vi "Overlord - MAIN - STARTUP.vi"(0 "Pathfinding Settings":T1={"Movement Settings"={"Arrival Tolerance (m)"=0.05, "Closeness Threshold (m)"=0.5, "Pit Obstacle Radius (m)"=0.4, "Pit Locations"=[]}, "Dead Zone"=0.9, "Max Moves"=4.0, "Move Segment Length (m)"=0.2, "Path Cost Weights"={"Length Weight"=1.0, "Angle Weight"=0.0, "Angle Error Weight"=75.0, "Angle Error Threshold"=1.04, "Per Move Penalty"=0.25, "Closeness Weight"=3.0, "Too Short Penalty"=100.0, "Too Short Threshold"=1.75}, "Desperation - Reduction Per Attempt (Ratio)"=0.9, "Desperation - Max Attempts"=2, "Log All Move Points"=FALSE, "Intermediate Position Grids"=[{"x1"=0.0, "x2"=4.75, "resolution"=0.45}]}) -> ()   [LabVIEW 2015, in "Overlord2017.lvlib"]
doc: "Note: pathfinding settings not required. This VI can run headless. Set default values before deploying to myRIO."
uses:
  Overlord2017.lvlib
  PathfindingSettings.ctl
  MovementSettings.ctl
  PathCostWeights.ctl
  IntermediatePositionGrids.ctl
  SubVIs - Overlord2017.lvlib
  TestbenchUtils - Navigation2017.lvlib
  Navigation2017.lvlib
  <vilib>/myRIO/Common/Instrument Driver Framework/Utilities/typedefs/Analog Scaling Constants.ctl
  <vilib>/myRIO/Common/Instrument Driver Framework/Utilities/typedefs/Analog Scaling Constants List.ctl
  <vilib>/myRIO/Common/Instrument Driver Framework/myRIO v1.0/AI/typedefs/AI Channels Enum.ctl
  <vilib>/myRIO/Common/Instrument Driver Framework/myRIO v1.0/AI/typedefs/AI Channels List.ctl
  <vilib>/myRIO/Common/Instrument Driver Framework/Utilities/typedefs/Generic FPGA Reference.ctl
  <vilib>/myRIO/Common/Instrument Driver Framework/Utilities/typedefs/myRIO v1.0 Reference.ctl
  <vilib>/myRIO/Common/Instrument Driver Framework/Utilities/typedefs/Hardware Version Enum.ctl
  <vilib>/myRIO/Common/Instrument Driver Framework/Utilities/typedefs/myRIO Generic Hardware Reference.ctl
  <vilib>/myRIO/Instrument Drivers/Onboard IO/AI/typedefs/AI Reference.ctl
  <vilib>/myRIO/Instrument Drivers/Onboard IO/AI/AI.lvlib
  <vilib>/myRIO/Instrument Drivers/Onboard IO/AI/vis/Read.vi
  <vilib>/myRIO/Instrument Drivers/Onboard IO/AI/vis/myRIO AI Open.xnode
  <vilib>/myRIO/Common/Instrument Driver Framework/Utilities/vis/Is FPGA Ref Available.vi
  <vilib>/myRIO/Express VI/Onboard IO/AI/AI Express VI.xnode
  <vilib>/myRIO/Common/Instrument Driver Framework/myRIO v1.0/AI/vis/myRIO v1.1 Open AI.vi
  <vilib>/userdefined/High Color/nirio_resource_hc.ctl
  Types - Navigation2017.lvlib
panel:
  out "Battery Voltage Chart":dbl(graph)=11.904298094
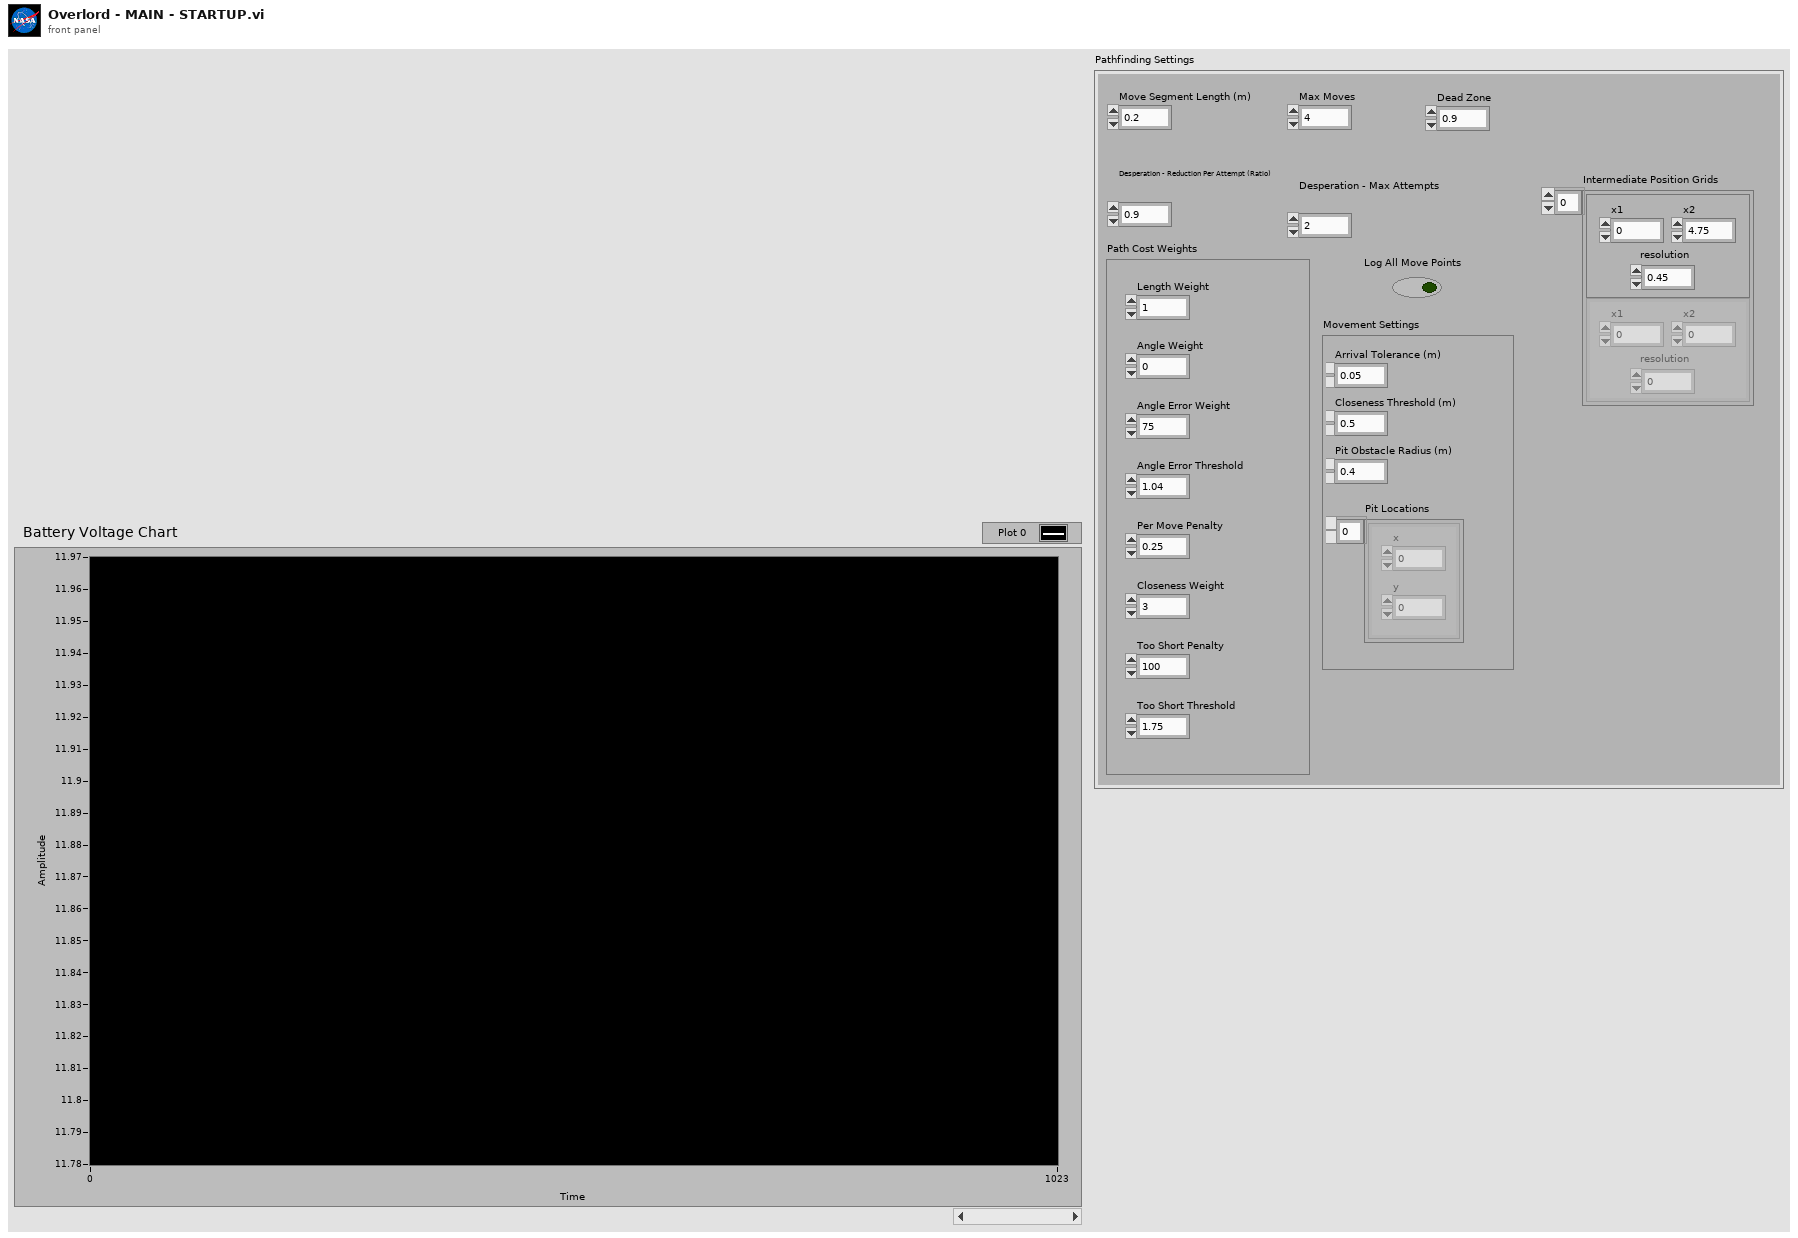
[diagram p1: front panel]
types:
  T1 = typedef "Navigation2017.lvlib/Types - Navigation2017.lvlib/PathfindingSettings.ctl" = cluster{"Movement Settings":T2, "Dead Zone":dbl, "Max Moves":dbl, "Move Segment Length (m)":dbl, "Path Cost Weights":T3, "Desperation - Reduction Per Attempt (Ratio)":dbl, "Desperation - Max Attempts":i16, "Log All Move Points":bool, "Intermediate Position Grids":T4}
  T2 = typedef "Navigation2017.lvlib/Types - Navigation2017.lvlib/MovementSettings.ctl" = cluster{"Arrival Tolerance (m)":dbl, "Closeness Threshold (m)":dbl, "Pit Obstacle Radius (m)":dbl, "Pit Locations":cluster{"x":dbl, "y":dbl}[]}
  T3 = typedef "Navigation2017.lvlib/Types - Navigation2017.lvlib/PathCostWeights.ctl" = cluster{"Length Weight":dbl, "Angle Weight":dbl, "Angle Error Weight":dbl, "Angle Error Threshold":dbl, "Per Move Penalty":dbl, "Closeness Weight":dbl, "Too Short Penalty":dbl, "Too Short Threshold":dbl}
  T4 = typedef "Navigation2017.lvlib/Types - Navigation2017.lvlib/IntermediatePositionGrids.ctl" = cluster{"x1":dbl, "x2":dbl, "resolution":dbl}[]
  T5 = typedef "AI.lvlib/AI Reference.ctl" = cluster{"myRIO Reference":T6, "AI Channels List":T10, "AI Scaling Constants List":T12}
  T6 = typedef "myRIO Generic Hardware Reference.ctl" = cluster{"myRIO Model":T7, "myRIO Hardware Reference":T8}
  T7 = typedef "Hardware Version Enum.ctl" = enum16{"Unknown", "myRIO-1900", "myRIO-1950", "roboRIO"}
  T8 = typedef "myRIO v1.0 Reference.ctl" = cluster{"Generic FPGA Reference":T9, "Allow multiple opens":bool}
  T9 = typedef "Generic FPGA Reference.ctl" = refnum<k20>
  T10 = typedef "AI Channels List.ctl" = T11[]
  T11 = typedef "AI Channels Enum.ctl" = enum16{"Not Connected", "AudioIn/Left", "AudioIn/Right", "C/AI0", "C/AI1", "A/AI0", "A/AI1", "A/AI2", "A/AI3", "B/AI0", "B/AI1", "B/AI2", "B/AI3", "AI/AI0", "AI/AI1", "AI/AI2", "AI/AI3"}
  T12 = typedef "Analog Scaling Constants List.ctl" = T13[]
  T13 = typedef "Analog Scaling Constants.ctl" = cluster{"LSB Weight (Volts)":dbl, "Offset (Volts)":dbl, "Signed?":bool}
  T14 = typedef "nirio_resource_hc.ctl" = tag
  T15 = enum16{"Spin and Move To Mining Area", "Move To Collector Trough", "Move To Mining Area"}
  T16 = typedef "Navigation2017.lvlib/TestbenchUtils - Navigation2017.lvlib/LocalizationStatus.ctl" = cluster{"x":dbl, "y":dbl, "angle":dbl, "valid":bool, "lastUpdatedTime":dbl}
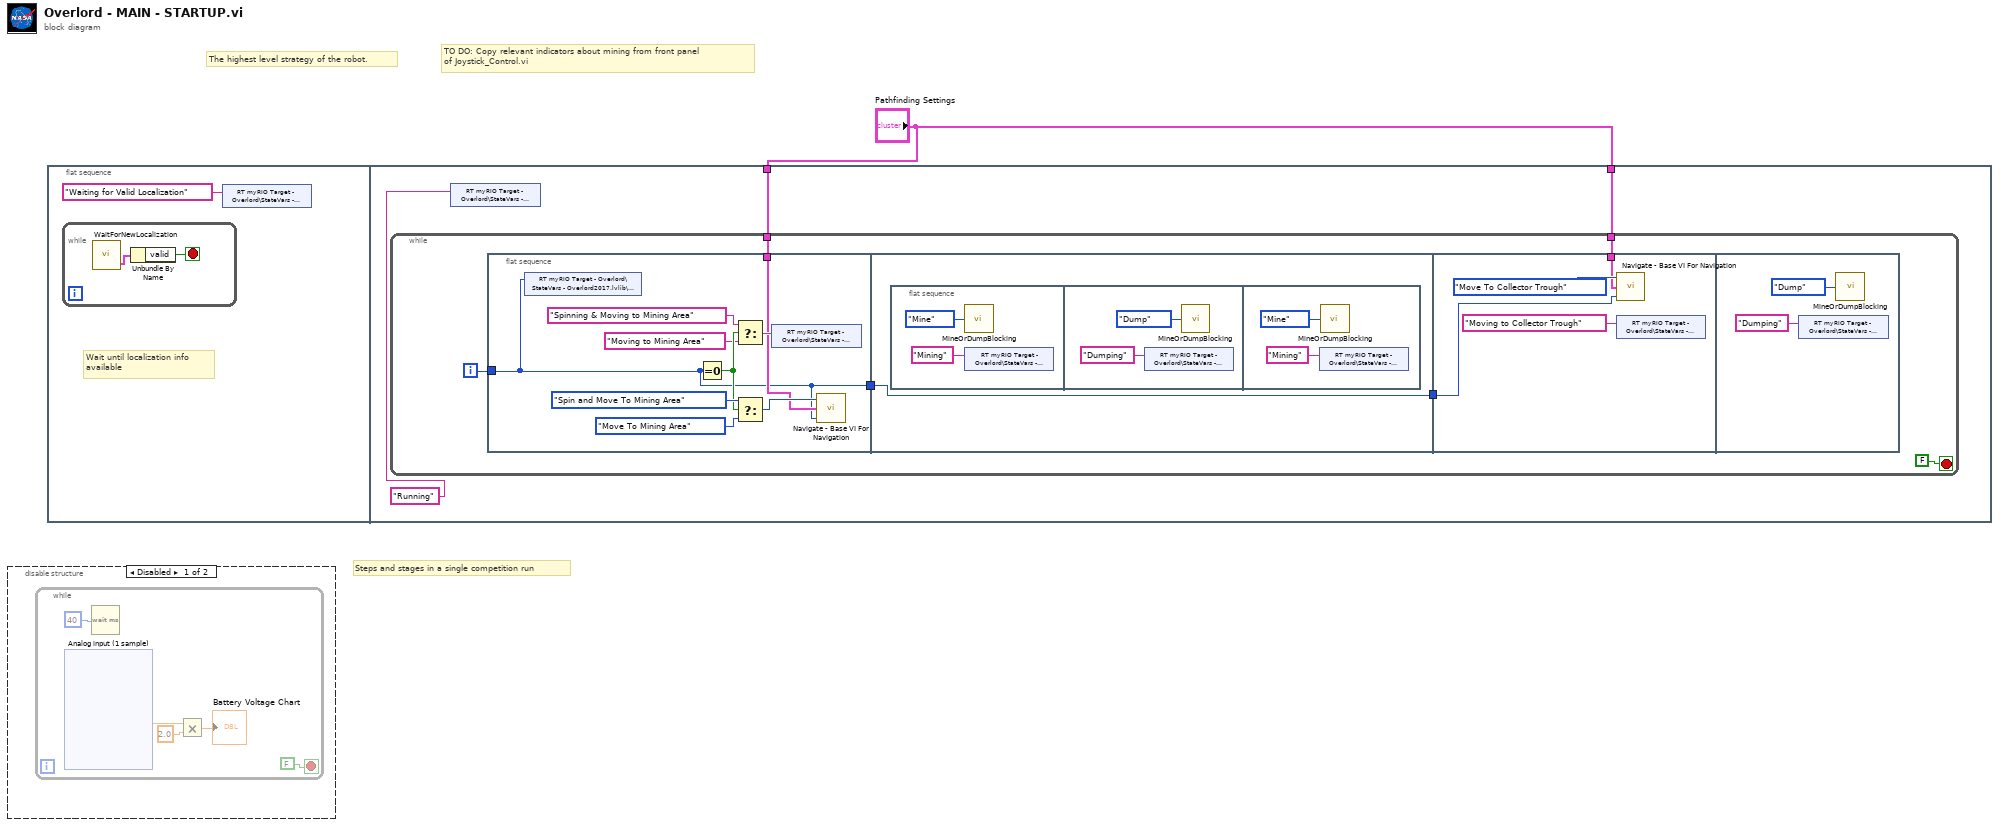
[diagram p0: block diagram]
diagram:
  # "The highest level strategy of the robot."
  # "Steps and stages in a single competition run"
  # "TO DO: Copy relevant indicators about mining from front panel\nof Joystick_Control.vi"
  n1 = disable-structure shown="Disabled" {
    frame Disabled {
      n2 = while {
        stop <- FALSE stop-if-true
        n3 = xnode "Analog input (1 sample)"() -> ("C/AI0 (AI0)"=w3:dbl)  [unwired: 1 in, 1 out]
        n4 = Wait (ms)(milliseconds to wait=u32 40) -> ()  [unwired: 1 out]
        n5 = Multiply(x=w3, y=2.0) -> (x*y=→"Battery Voltage Chart":dbl)
      }
    }
    frame Enabled {
    }
  }
  n6 = flat-sequence {
    tunnel: "Pathfinding Settings" -> [w48]
    tunnel: "Pathfinding Settings" -> [w47]
    frame #0 {
      # "Wait until localization info\navailable"
      n7 = while {
        stop <- w46 stop-if-true
        n8 = call "WaitForNewLocalization.vi"() -> ("Localization Status"=w45:T16)  [unwired: 1 out]
        n9 = Unbundle By Name(w45) -> ("valid"=w46:bool)
      }
      n10 = shared-variable "RT myRIO Target - Overlord\\StateVars - Overlord2017.lvlib\\CurrStage"("Waiting for Valid Localization" ("CurrStage")) -> ()  [unwired: 1 in, 1 out]
    }
    frame #1 {
      n11 = while {
        tunnel: w48 -> [w53]
        tunnel: w47 -> [w52]
        i -> [w55]
        stop <- FALSE stop-if-true
        n12 = flat-sequence {
          tunnel: w55 -> [w56]
          tunnel: w53 -> [w57]
          tunnel: [w56] -> w51
          tunnel: w51 -> [w65]
          tunnel: [w65] -> w50
          tunnel: w52 -> [w73]
          tunnel: w50 -> [w72]
          frame #0 {
            n13 = shared-variable "RT myRIO Target - Overlord\\StateVars - Overlord2017.lvlib\\CurrMiningRun"(w56) -> ()  [unwired: 1 in, 1 out]
            n14 = Equal To 0?(x=w56) -> (x = 0?=w59:bool)
            n15 = Select(t="Spinning & Moving to Mining Area" ("CurrStage"), s=w59, f="Moving to Mining Area") -> (s? t:f=w61:string)
            n16 = Select(t=T15."Spin and Move To Mining Area" ("Move Type"), s=w59, f=T15."Move To Mining Area") -> (s? t:f=w62:T15)
            n17 = shared-variable "RT myRIO Target - Overlord\\StateVars - Overlord2017.lvlib\\CurrStage"(w61) -> ()  [unwired: 1 in, 1 out]
            n18 = call "Navigate - Base VI For Navigation.vi"("Curr Mining Run"=w56, "Pathfinding Settings"=w57, "Move Type"=w62) -> ()  [unwired: 1 in]
          }
          frame #1 {
            n19 = flat-sequence {
              frame #0 {
                n20 = call "MineOrDumpBlocking.vi"("Action"=enum16{"Dump", "Mine"}."Mine") -> ()
                n21 = shared-variable "RT myRIO Target - Overlord\\StateVars - Overlord2017.lvlib\\CurrStage"("Mining" ("CurrStage")) -> ()  [unwired: 1 in, 1 out]
              }
              frame #1 {
                n22 = shared-variable "RT myRIO Target - Overlord\\StateVars - Overlord2017.lvlib\\CurrStage"("Dumping" ("CurrStage")) -> ()  [unwired: 1 in, 1 out]
                n23 = call "MineOrDumpBlocking.vi"("Action"=enum16{"Dump", "Mine"}."Dump") -> ()
              }
              frame #2 {
                n24 = shared-variable "RT myRIO Target - Overlord\\StateVars - Overlord2017.lvlib\\CurrStage"("Mining" ("CurrStage")) -> ()  [unwired: 1 in, 1 out]
                n25 = call "MineOrDumpBlocking.vi"("Action"=enum16{"Dump", "Mine"}."Mine") -> ()
              }
            }
          }
          frame #2 {
            n26 = call "Navigate - Base VI For Navigation.vi"("Curr Mining Run"=w72, "Pathfinding Settings"=w73, "Move Type"=T15."Move To Collector Trough") -> ()  [unwired: 1 in]
            n27 = shared-variable "RT myRIO Target - Overlord\\StateVars - Overlord2017.lvlib\\CurrStage"("Moving to Collector Trough" ("CurrStage")) -> ()  [unwired: 1 in, 1 out]
          }
          frame #3 {
            n28 = shared-variable "RT myRIO Target - Overlord\\StateVars - Overlord2017.lvlib\\CurrStage"("Dumping" ("CurrStage")) -> ()  [unwired: 1 in, 1 out]
            n29 = call "MineOrDumpBlocking.vi"("Action"=enum16{"Dump", "Mine"}."Dump") -> ()
          }
        }
      }
      n30 = shared-variable "RT myRIO Target - Overlord\\StateVars - Overlord2017.lvlib\\CurrStage"("Running" ("CurrStage")) -> ()  [unwired: 1 in, 1 out]
    }
  }
